vi "add_elementToAgents_p.vi"(0 "MoAgSy_Host":refnum<class "MoAgSy_Host.lvclass">, 3 "Agent ID":string, 5 "error in (no error)":errorcluster) -> (14 "dup MoAgSy_Host":refnum<class "MoAgSy_Host.lvclass">, 19 "error out":errorcluster)   [LabVIEW 2009, in "MoAgSy.lvlib" / "MoAgSy_Host.lvclass"]
doc: "<B>protected</B> VI adds new started agents id to mobile agent host classes running agents list.\nIs called by public add element to Agents VI\n\nF.Berck@gsi.de\nGSI Darmstadt 2009"
uses:
  MoAgSy_Host.lvclass
  MoAgSy_Host.lvclass/MoAgSy_Host.ctl
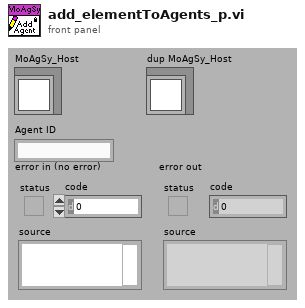
[diagram p1: front panel]
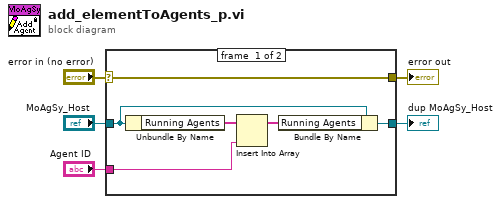
[diagram p0: block diagram]
diagram:
  n1 = case shown="No Error" "error in (no error)" {
    selector: "error in (no error)" -> [w11 w12]
    tunnel: [w11 w12] -> w4
    tunnel: [w10 w13] -> w2
    tunnel: "MoAgSy_Host" -> [w9 w13]
    tunnel: "Agent ID" -> [w6 _]
    frame #0 {
      n2 = Unbundle By Name(w9) -> ("Running Agents"=w8:string[])
      n3 = Insert Into Array(array=w8, new element=w6) -> (w7:string[])  [unwired: 1 in]
      n4 = Bundle By Name(cluster=w9, "Running Agents"=w7) -> (w10:refnum<class "MoAgSy_Host.lvclass">)
    }
    frame #1 {
    }
  }
  "error out" <- w4
  "dup MoAgSy_Host" <- w2
